vi "Scoreboard(SubVI).vi"(0 "Boolean (Eingang)":refnum<vi>, 1 "Tic Tac Toe (Eingang)":u8[][](array[numeric]), 2 "Leicht":T1, 3 "Enum":T3(ring), 5 "Mittel":T1, 7 "Unmöglich":T1, 9 "Mit Fruende":T1, 11 "Next Turn":i8, 12 "DateSpeicherPath":path, 14 "Ergebnis":bool) -> (4 "Score 5":T2, 6 "Score 6":T2, 8 "Score 7":T2, 10 "Score 8":T2)   [LabVIEW 2017]
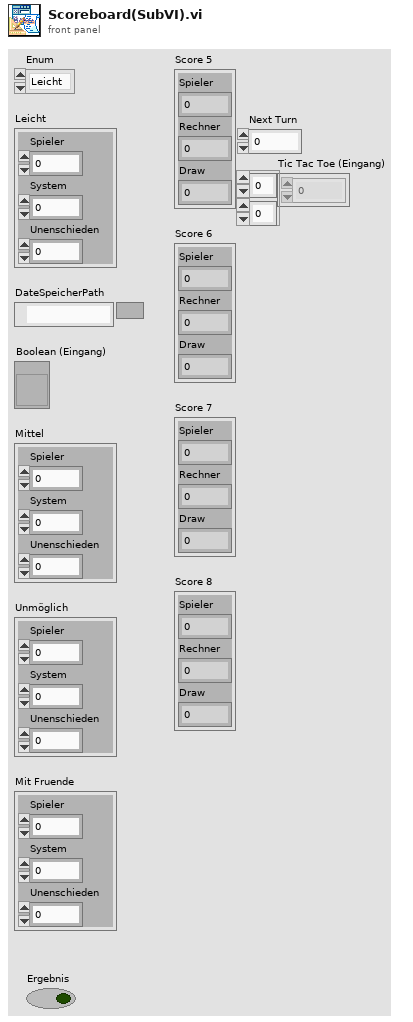
[diagram p1: front panel]
types:
  T1 = cluster{"Spieler":u32, "System":u32, "Unenschieden":u32}
  T2 = cluster{"Spieler":dbl, "Rechner":dbl, "Draw":dbl}
  T3 = enum16{"Leicht", "Mittel", "Unmöglich", "Mit einem Freund Spielen"}
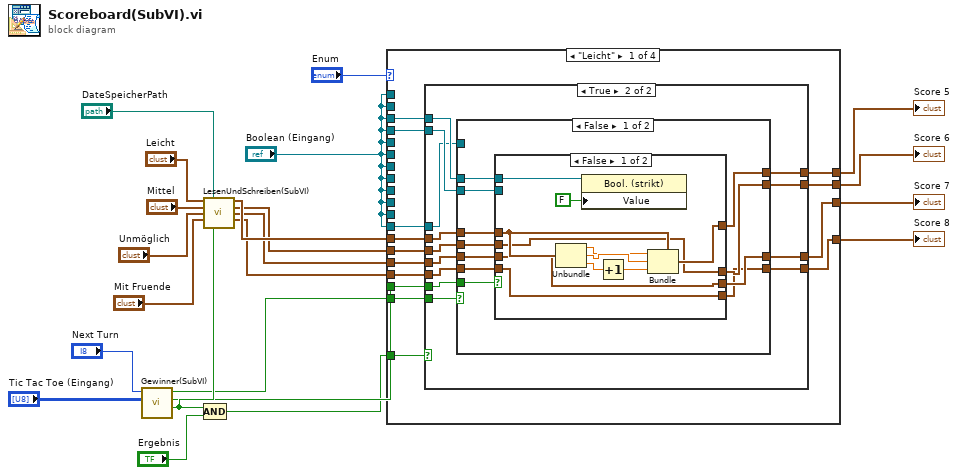
[diagram p0: block diagram]
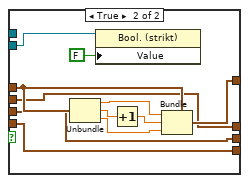
[diagram p3: hidden frame]
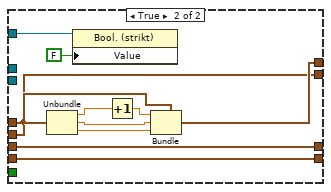
[diagram p4: hidden frame]
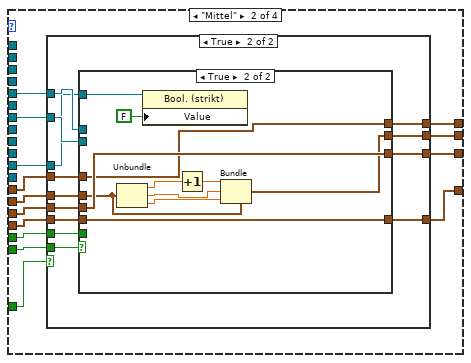
[diagram p5: hidden frame]
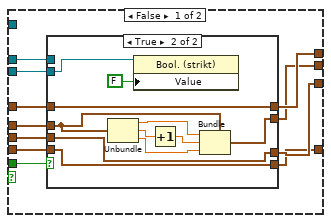
[diagram p7: hidden frame]
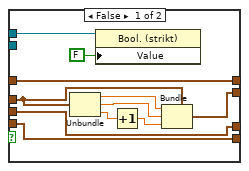
[diagram p8: hidden frame]
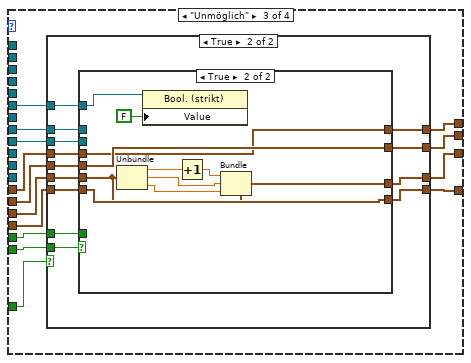
[diagram p9: hidden frame]
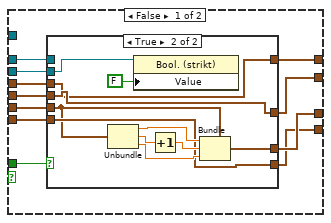
[diagram p11: hidden frame]
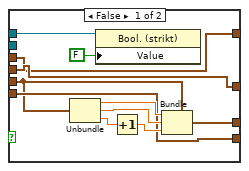
[diagram p12: hidden frame]
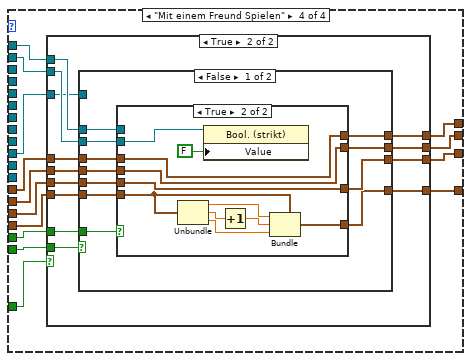
[diagram p13: hidden frame]
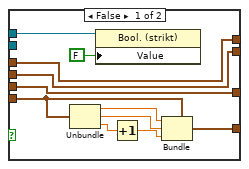
[diagram p15: hidden frame]
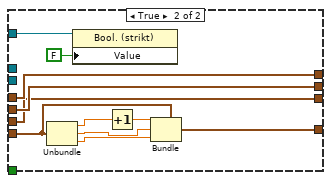
[diagram p16: hidden frame]
diagram:
  n1 = call "Gewinner(SubVI).vi"("Array"="Tic Tac Toe (Eingang)", "Next Turn"="Next Turn") -> ("Game over"=w20:bool, "Win 2"=w19:bool, "Win"=w18:bool)  [unwired: 7 in]
  n2 = call "LesenUndSchreiben(SubVI).vi"("Score"="Leicht", "file path (dialog if empty)"="DateSpeicherPath", "Score 2"="Mittel", "Score 3"="Unmöglich", "Score 4"="Mit Fruende", "gameOver"=w20) -> ("Score 5"=w11:T2, "Score 6"=w10:T2, "Score 7"=w9:T2, "Score 8"=w8:T2)  [unwired: 6 in]
  n3 = Compound Arithmetic op=AND ("Mehrfacharithmetik")(w20, "Ergebnis") -> (w2:bool)
  n4 = case shown="\"Leicht\"" "Enum" {
    tunnel: w2 -> [w36 w111 w186 w261]
    tunnel: w11 -> [w35 w110 w185 w260]
    tunnel: w10 -> [w34 w109 w184 w259]
    tunnel: w9 -> [w33 w108 w183 w258]
    tunnel: w8 -> [w32 w107 w182 w257]
    tunnel: w18 -> [w26 w106 w181 w251]
    tunnel: w19 -> [w31 w105 w180 w256]
    tunnel: [w30 w104 w179 w255] -> w6
    tunnel: [w29 w103 w178 w254] -> w5
    tunnel: [w28 w102 w177 w253] -> w4
    tunnel: [w27 w101 w176 w252] -> w3
    tunnel: "Boolean (Eingang)" -> [w25 _ _ _]
    tunnel: "Boolean (Eingang)" -> [w24 _ _ _]
    tunnel: "Boolean (Eingang)" -> [w23 _ _ _]
    tunnel: "Boolean (Eingang)" -> [_ w100 _ _]
    tunnel: "Boolean (Eingang)" -> [_ w99 _ _]
    tunnel: "Boolean (Eingang)" -> [_ w98 _ _]
    tunnel: "Boolean (Eingang)" -> [_ _ w175 _]
    tunnel: "Boolean (Eingang)" -> [_ _ w174 _]
    tunnel: "Boolean (Eingang)" -> [_ _ w173 _]
    tunnel: "Boolean (Eingang)" -> [_ _ _ w250]
    tunnel: "Boolean (Eingang)" -> [_ _ _ w249]
    tunnel: "Boolean (Eingang)" -> [_ _ _ w248]
    frame "Leicht" {
      n5 = case shown="True" w36 {
        tunnel: w35 -> [w40 w53]
        tunnel: w34 -> [w39 w51]
        tunnel: w33 -> [w38 w50]
        tunnel: w32 -> [w37 w49]
        tunnel: [w40 w52] -> w30
        tunnel: w31 -> [_ w48]
        tunnel: [w39 w47] -> w29
        tunnel: [w38 w44] -> w28
        tunnel: [w37 w46] -> w27
        tunnel: w26 -> [_ w45]
        tunnel: w25 -> [_ w43]
        tunnel: w24 -> [_ w42]
        tunnel: w23 -> [_ w41]
        frame False {
        }
        frame True {
          n6 = case shown="False" w45 {
            tunnel: w53 -> [w64 w92]
            tunnel: [w59 w97] -> w52
            tunnel: w51 -> [w63 w91]
            tunnel: w50 -> [w62 w90]
            tunnel: w49 -> [w61 w89]
            tunnel: w48 -> [w60 _]
            tunnel: [w58 w91] -> w47
            tunnel: [w57 w90] -> w44
            tunnel: [w56 w89] -> w46
            tunnel: w43 -> [w55 _]
            tunnel: w42 -> [w54 _]
            tunnel: w41 -> [_ w87]
            frame False {
              n7 = case shown="False" w60 {
                tunnel: w64 -> [w73 w85]
                tunnel: w63 -> [w69 w80]
                tunnel: w62 -> [w68 w79]
                tunnel: w61 -> [w67 w78]
                tunnel: [w74 w81] -> w59
                tunnel: [w69 w80] -> w58
                tunnel: [w68 w79] -> w57
                tunnel: [w67 w78] -> w56
                tunnel: w55 -> [w65 _]
                tunnel: w54 -> [_ w76]
                frame False {
                  n8 = Unbundle(w73) -> ("Spieler"=w70:dbl, "Rechner"=w75:dbl, "Draw"=w72:dbl)
                  n9 = property class="Bool. (strikt)"(reference=w65, "Value"=FALSE) -> ()  [unwired: 1 in, 2 out]
                  n10 = Increment(x=w72) -> (x+1=w71:dbl)
                  n11 = Bundle(cluster=w73, "Spieler"=w70, "Rechner"=w75, "Draw"=w71) -> (w74:T2)
                }
                frame True {
                  n12 = Unbundle(w85) -> ("Spieler"=w83:dbl, "Rechner"=w82:dbl, "Draw"=w86:dbl)
                  n13 = property class="Bool. (strikt)"(reference=w76, "Value"=FALSE) -> ()  [unwired: 1 in, 2 out]
                  n14 = Increment(x=w82) -> (x+1=w84:dbl)
                  n15 = Bundle(cluster=w85, "Spieler"=w83, "Rechner"=w84, "Draw"=w86) -> (w81:T2)
                }
              }
            }
            frame True {
              n16 = Unbundle(w92) -> ("Spieler"=w96:dbl, "Rechner"=w94:dbl, "Draw"=w93:dbl)
              n17 = property class="Bool. (strikt)"(reference=w87, "Value"=FALSE) -> ()  [unwired: 1 in, 2 out]
              n18 = Increment(x=w96) -> (x+1=w95:dbl)
              n19 = Bundle(cluster=w92, "Spieler"=w95, "Rechner"=w94, "Draw"=w93) -> (w97:T2)
            }
          }
        }
      }
    }
    frame "Mittel" {
      n20 = case shown="True" w111 {
        tunnel: w110 -> [w115 w128]
        tunnel: w109 -> [w114 w126]
        tunnel: w108 -> [w113 w125]
        tunnel: w107 -> [w112 w124]
        tunnel: [w115 w127] -> w104
        tunnel: w106 -> [_ w123]
        tunnel: w105 -> [_ w122]
        tunnel: [w114 w121] -> w103
        tunnel: [w113 w120] -> w102
        tunnel: [w112 w119] -> w101
        tunnel: w100 -> [_ w118]
        tunnel: w99 -> [_ w117]
        tunnel: w98 -> [_ w116]
        frame False {
        }
        frame True {
          n21 = case shown="True" w123 {
            tunnel: w128 -> [w139 w164]
            tunnel: [w134 w164] -> w127
            tunnel: w126 -> [w138 w166]
            tunnel: w125 -> [w137 w168]
            tunnel: w124 -> [w136 w167]
            tunnel: w122 -> [w135 _]
            tunnel: [w133 w165] -> w121
            tunnel: [w132 w168] -> w120
            tunnel: [w131 w167] -> w119
            tunnel: w118 -> [w130 _]
            tunnel: w117 -> [w129 _]
            tunnel: w116 -> [_ w162]
            frame False {
              n22 = case shown="True" w135 {
                tunnel: w139 -> [w142 w153]
                tunnel: w138 -> [w143 w155]
                tunnel: w137 -> [w146 w157]
                tunnel: w136 -> [w145 w156]
                tunnel: [w142 w153] -> w134
                tunnel: [w144 w154] -> w133
                tunnel: [w146 w157] -> w132
                tunnel: [w145 w156] -> w131
                tunnel: w130 -> [w140 _]
                tunnel: w129 -> [_ w151]
                frame False {
                  n23 = Unbundle(w143) -> ("Spieler"=w147:dbl, "Rechner"=w150:dbl, "Draw"=w149:dbl)
                  n24 = property class="Bool. (strikt)"(reference=w140, "Value"=FALSE) -> ()  [unwired: 1 in, 2 out]
                  n25 = Increment(x=w149) -> (x+1=w148:dbl)
                  n26 = Bundle(cluster=w143, "Spieler"=w147, "Rechner"=w150, "Draw"=w148) -> (w144:T2)
                }
                frame True {
                  n27 = Unbundle(w155) -> ("Spieler"=w159:dbl, "Rechner"=w158:dbl, "Draw"=w161:dbl)
                  n28 = property class="Bool. (strikt)"(reference=w151, "Value"=FALSE) -> ()  [unwired: 1 in, 2 out]
                  n29 = Increment(x=w158) -> (x+1=w160:dbl)
                  n30 = Bundle(cluster=w155, "Spieler"=w159, "Rechner"=w160, "Draw"=w161) -> (w154:T2)
                }
              }
            }
            frame True {
              n31 = Unbundle(w166) -> ("Spieler"=w172:dbl, "Rechner"=w170:dbl, "Draw"=w169:dbl)
              n32 = property class="Bool. (strikt)"(reference=w162, "Value"=FALSE) -> ()  [unwired: 1 in, 2 out]
              n33 = Increment(x=w172) -> (x+1=w171:dbl)
              n34 = Bundle(cluster=w166, "Spieler"=w171, "Rechner"=w170, "Draw"=w169) -> (w165:T2)
            }
          }
        }
      }
    }
    frame "Unmöglich" {
      n35 = case shown="True" w186 {
        tunnel: w185 -> [w187 w203]
        tunnel: w184 -> [w190 w201]
        tunnel: w183 -> [w189 w200]
        tunnel: w182 -> [w188 w199]
        tunnel: [w187 w202] -> w179
        tunnel: w181 -> [_ w198]
        tunnel: w180 -> [_ w197]
        tunnel: [w190 w196] -> w178
        tunnel: [w189 w195] -> w177
        tunnel: [w188 w194] -> w176
        tunnel: w175 -> [_ w193]
        tunnel: w174 -> [_ w192]
        tunnel: w173 -> [_ w191]
        frame False {
        }
        frame True {
          n36 = case shown="True" w198 {
            tunnel: w203 -> [w214 w239]
            tunnel: [w209 w239] -> w202
            tunnel: w201 -> [w213 w243]
            tunnel: w200 -> [w212 w241]
            tunnel: w199 -> [w211 w242]
            tunnel: w197 -> [w210 _]
            tunnel: [w208 w243] -> w196
            tunnel: [w207 w240] -> w195
            tunnel: [w206 w242] -> w194
            tunnel: w193 -> [w205 _]
            tunnel: w192 -> [w204 _]
            tunnel: w191 -> [_ w237]
            frame False {
              n37 = case shown="True" w210 {
                tunnel: w214 -> [w217 w228]
                tunnel: w213 -> [w221 w232]
                tunnel: w212 -> [w218 w229]
                tunnel: w211 -> [w220 w231]
                tunnel: [w217 w228] -> w209
                tunnel: [w221 w232] -> w208
                tunnel: [w219 w230] -> w207
                tunnel: [w220 w231] -> w206
                tunnel: w205 -> [w215 _]
                tunnel: w204 -> [_ w226]
                frame False {
                  n38 = Unbundle(w218) -> ("Spieler"=w222:dbl, "Rechner"=w225:dbl, "Draw"=w224:dbl)
                  n39 = property class="Bool. (strikt)"(reference=w215, "Value"=FALSE) -> ()  [unwired: 1 in, 2 out]
                  n40 = Increment(x=w224) -> (x+1=w223:dbl)
                  n41 = Bundle(cluster=w218, "Spieler"=w222, "Rechner"=w225, "Draw"=w223) -> (w219:T2)
                }
                frame True {
                  n42 = Unbundle(w229) -> ("Spieler"=w234:dbl, "Rechner"=w233:dbl, "Draw"=w236:dbl)
                  n43 = property class="Bool. (strikt)"(reference=w226, "Value"=FALSE) -> ()  [unwired: 1 in, 2 out]
                  n44 = Increment(x=w233) -> (x+1=w235:dbl)
                  n45 = Bundle(cluster=w229, "Spieler"=w234, "Rechner"=w235, "Draw"=w236) -> (w230:T2)
                }
              }
            }
            frame True {
              n46 = Unbundle(w241) -> ("Spieler"=w247:dbl, "Rechner"=w245:dbl, "Draw"=w244:dbl)
              n47 = property class="Bool. (strikt)"(reference=w237, "Value"=FALSE) -> ()  [unwired: 1 in, 2 out]
              n48 = Increment(x=w247) -> (x+1=w246:dbl)
              n49 = Bundle(cluster=w241, "Spieler"=w246, "Rechner"=w245, "Draw"=w244) -> (w240:T2)
            }
          }
        }
      }
    }
    frame "Mit einem Freund Spielen" {
      n50 = case shown="True" w261 {
        tunnel: w260 -> [w265 w278]
        tunnel: w259 -> [w264 w276]
        tunnel: w258 -> [w263 w275]
        tunnel: w257 -> [w262 w274]
        tunnel: [w265 w277] -> w255
        tunnel: w256 -> [_ w273]
        tunnel: [w264 w272] -> w254
        tunnel: [w263 w271] -> w253
        tunnel: [w262 w270] -> w252
        tunnel: w251 -> [_ w269]
        tunnel: w250 -> [_ w268]
        tunnel: w249 -> [_ w267]
        tunnel: w248 -> [_ w266]
        frame False {
        }
        frame True {
          n51 = case shown="False" w269 {
            tunnel: w278 -> [w289 w316]
            tunnel: [w284 w316] -> w277
            tunnel: w276 -> [w288 w318]
            tunnel: w275 -> [w287 w315]
            tunnel: w274 -> [w286 w317]
            tunnel: w273 -> [w285 _]
            tunnel: [w283 w318] -> w272
            tunnel: [w282 w315] -> w271
            tunnel: [w281 w314] -> w270
            tunnel: w268 -> [w280 _]
            tunnel: w267 -> [w279 _]
            tunnel: w266 -> [_ w312]
            frame False {
              n52 = case shown="True" w285 {
                tunnel: w289 -> [w292 w303]
                tunnel: w288 -> [w296 w307]
                tunnel: w287 -> [w295 w306]
                tunnel: w286 -> [w294 w305]
                tunnel: [w292 w303] -> w284
                tunnel: [w296 w307] -> w283
                tunnel: [w295 w306] -> w282
                tunnel: [w293 w304] -> w281
                tunnel: w280 -> [w290 _]
                tunnel: w279 -> [_ w301]
                frame False {
                  n53 = Unbundle(w294) -> ("Spieler"=w297:dbl, "Rechner"=w300:dbl, "Draw"=w299:dbl)
                  n54 = property class="Bool. (strikt)"(reference=w290, "Value"=FALSE) -> ()  [unwired: 1 in, 2 out]
                  n55 = Increment(x=w299) -> (x+1=w298:dbl)
                  n56 = Bundle(cluster=w294, "Spieler"=w297, "Rechner"=w300, "Draw"=w298) -> (w293:T2)
                }
                frame True {
                  n57 = Unbundle(w305) -> ("Spieler"=w309:dbl, "Rechner"=w308:dbl, "Draw"=w311:dbl)
                  n58 = property class="Bool. (strikt)"(reference=w301, "Value"=FALSE) -> ()  [unwired: 1 in, 2 out]
                  n59 = Increment(x=w308) -> (x+1=w310:dbl)
                  n60 = Bundle(cluster=w305, "Spieler"=w309, "Rechner"=w310, "Draw"=w311) -> (w304:T2)
                }
              }
            }
            frame True {
              n61 = Unbundle(w317) -> ("Spieler"=w322:dbl, "Rechner"=w320:dbl, "Draw"=w319:dbl)
              n62 = property class="Bool. (strikt)"(reference=w312, "Value"=FALSE) -> ()  [unwired: 1 in, 2 out]
              n63 = Increment(x=w322) -> (x+1=w321:dbl)
              n64 = Bundle(cluster=w317, "Spieler"=w321, "Rechner"=w320, "Draw"=w319) -> (w314:T2)
            }
          }
        }
      }
    }
  }
  "Score 8" <- w3
  "Score 7" <- w4
  "Score 6" <- w5
  "Score 5" <- w6
